vi "Append Hypertext Link Anchor to Report.vi"(0 "report in":refnum<class "NI_HTML.lvclass">, 1 "MS Office parameters":T1, 5 "URL of link - href":string, 9 "link text":string, 11 "error in (no error)":errorcluster) -> (4 "report out":refnum<class "NI_HTML.lvclass">, 8 "start out (word)":i32, 10 "end out (word)":i32, 15 "error out":errorcluster)   [LabVIEW 2020, in "NI_HTML.lvclass"]
doc: "Creates and adds a hypertext link anchor to a Word, Excel, or HTML report. You cannot use this VI with standard reports."
uses:
  NI_HTML.lvclass
  NI_HTML.lvclass/NI_HTML.ctl
  NI_ReportGenerationCore.lvlib
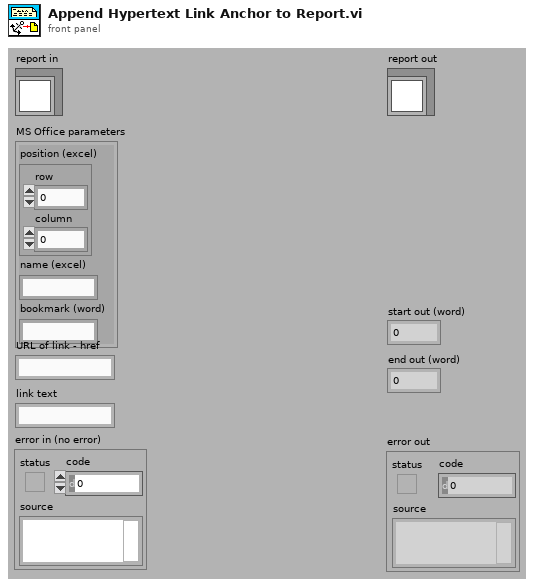
[diagram p1: front panel]
types:
  T1 = cluster{"position (excel)":cluster{"row":i32, "column":i32}, "name (excel)":string, "bookmark (word)":string}
  T2 = typedef "NI_ReportGenerationCore.lvlib/HTML Report Data.ctl" = cluster{"Body Text":string, "Font Tag":string, "Title Text":string, "Header Text":string, "Footer Text":string, "Image List":path[]}
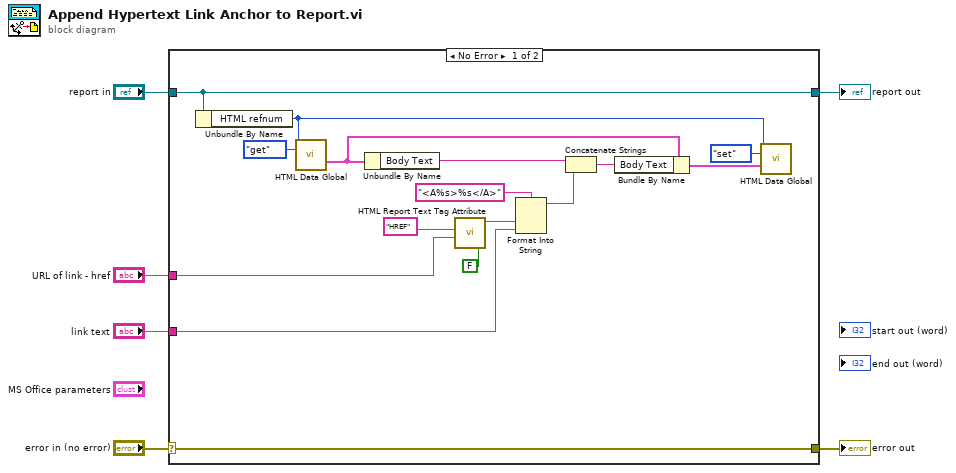
[diagram p0: block diagram]
diagram:
  n1 = case shown="No Error" "error in (no error)" {
    selector: "error in (no error)" -> [w22 w24]
    tunnel: [w22 w24] -> w5
    tunnel: [w12 w23] -> w3
    tunnel: "report in" -> [w12 w23]
    tunnel: "URL of link - href" -> [w16 _]
    tunnel: "link text" -> [w15 _]
    frame No Error {
      n2 = Unbundle By Name(w12) -> ("HTML refnum"=w7:u32)
      n3 = call "HTML Data Global.vi"("HTML refnum"=w7, "menu"=enum16{"init", "get", "set", "delete"}."get") -> ("HTML report data out"=w8:T2)  [unwired: 1 in, 12 out]
      n4 = Unbundle By Name(w8) -> ("Body Text"=w13:string)
      n5 = call "HTML Report Text Tag Attribute.vi"("filter value (T)"=FALSE ("escape value (T)"), "value"=w16, "label"="HREF") -> ("tag attributes out"=w21:string)  [unwired: 1 in, 3 out]
      n6 = Format Into String(format string="<A%s>%s</A>", w21, w15) -> (resulting string=w20:string)  [unwired: 2 in, 1 out]
      n7 = Concatenate Strings(w13, w20) -> (w9:string)
      n8 = Bundle By Name(cluster=w8, "Body Text"=w9) -> (w11:T2)
      n9 = call "HTML Data Global.vi"("HTML refnum"=w7, "menu"=enum16{"init", "get", "set", "delete"}."set", "HTML report data in"=w11) -> ()  [unwired: 13 out]
    }
    frame Error {
    }
  }
  "error out" <- w5
  "report out" <- w3
